vi "AI端口_行程.vi"() -> ()   [LabVIEW 2013]
panel:
  out "行程":tag="Dev1/ai0"
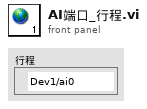
[diagram p1: front panel]
diagram:
